vi "WCM_state_change.vi"(8 "error in (no error)":errorcluster, 10 "WCM_state":T1, 11 "Control-Client in":refnum<class "Control-Client.lvclass">) -> (0 "error out":errorcluster, 3 "Control-Client out":refnum<class "Control-Client.lvclass">)   [LabVIEW 2019, in "Control-Client.lvclass"]
uses:
  Control-Client.lvclass
  controls/WCM.ctl
  dependecies/ControlsVIs/Clusters-def/SERVER-Commands.ctl
  dependecies/ControlsVIs/Clusters-def/Message types.ctl
  Control-Client.lvclass/Control-Client.ctl
  Control-Server/Control-Server.lvclass
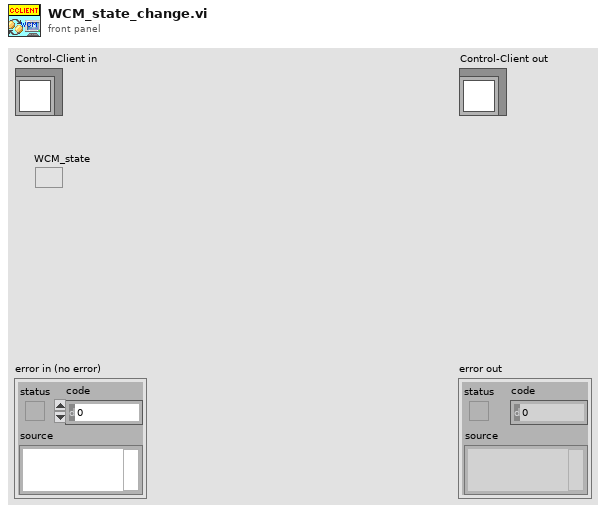
[diagram p1: front panel]
types:
  T1 = typedef "WCM.ctl" = bool
  T2 = typedef "Message types.ctl" = string
  T3 = typedef "Control-Server.lvclass/SERVER-Commands.ctl" = string
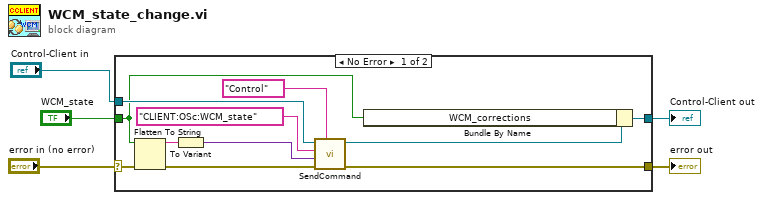
[diagram p0: block diagram]
diagram:
  n1 = case shown="No Error" "error in (no error)" {
    selector: "error in (no error)" -> [w16 w18]
    tunnel: [w15 w18] -> w4
    tunnel: [w7 w17] -> w2
    tunnel: "Control-Client in" -> [w14 w17]
    tunnel: "WCM_state" -> [w6 _]
    frame No Error {
      n2 = Flatten To String(anything=w6, error in (no error)=w16) -> (data string=w9:string, error out=w10:errorcluster)  [unwired: 2 in, 1 out]
      n3 = To Variant(anything=w9) -> (Variant=w12:variant)
      n4 = call "SendCommand.vi"("Message type"=T2 "Control", "error in (no error)"=w10, "data"=w12, "Command"=T3 "CLIENT:OSc:WCM_state" ("Commands"), "Control-Client in"=w14) -> ("error out"=w15:errorcluster, "Control-Client out"=w8:refnum<class "Control-Client.lvclass">)  [unwired: 5 in]
      n5 = Bundle By Name(cluster=w8, "WCM_corrections"=w6) -> (w7:refnum<class "Control-Client.lvclass">)
    }
    frame Error {
    }
  }
  "error out" <- w4
  "Control-Client out" <- w2
